vi "Initialize.vi"(0 "Socket Auto Connect in":refnum<class "Socket Auto Connect.lvclass">, 5 "error in (no error)":errorcluster) -> (14 "Socket Auto Connect out":refnum<class "Socket Auto Connect.lvclass">, 19 "error out":errorcluster)   [LabVIEW 2019, in "Socket Auto Connect.lvclass"]
uses:
  Socket Auto Connect.lvclass
  Socket Auto Connect.lvclass/Socket Auto Connect.ctl
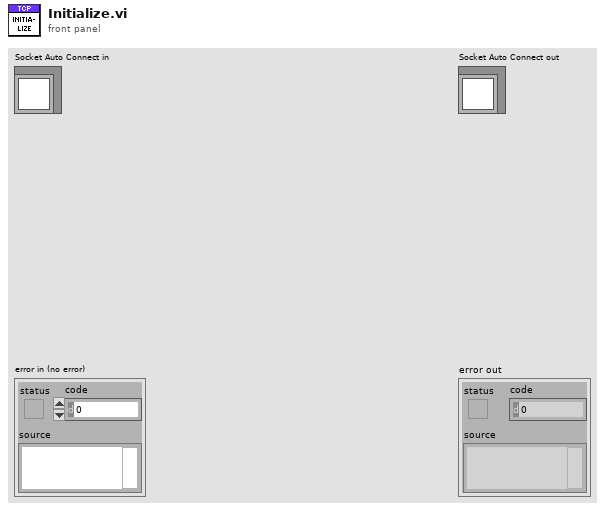
[diagram p1: front panel]
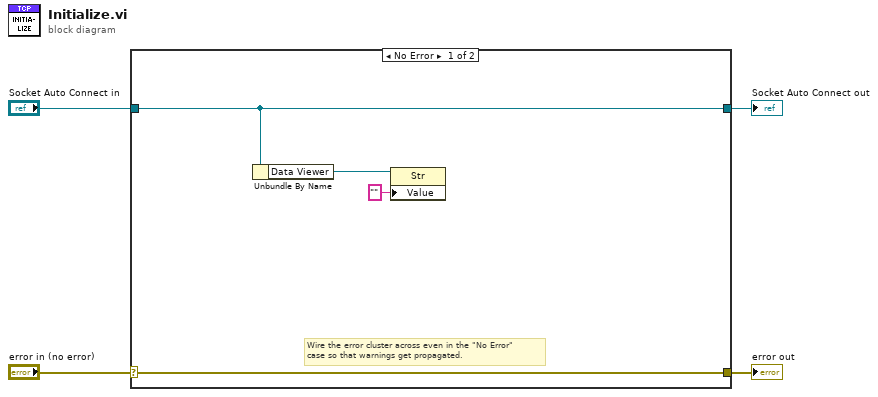
[diagram p0: block diagram]
diagram:
  n1 = case shown="No Error" "error in (no error)" {
    selector: "error in (no error)" -> [w8 w10]
    tunnel: [w8 w10] -> w3
    tunnel: [w7 w9] -> w1
    tunnel: "Socket Auto Connect in" -> [w7 w9]
    frame No Error {
      # "Wire the error cluster across even in the \"No Error\"\ncase so that warnings get propagated."
      n2 = Unbundle By Name(w7) -> ("Data Viewer"=w6:refnum<vi>)
      n3 = property class="Str"(reference=w6, "Value"="") -> ()  [unwired: 1 in, 2 out]
    }
    frame Error {
    }
  }
  "error out" <- w3
  "Socket Auto Connect out" <- w1
